vi "CreateCreepSamples2.vi"(0 "setValueForAESum":dbl, 5 "AEdataSum":dbl, 7 "outputLength":i32, 9 "changeOfForceWithinBufferLoop":dbl, 11 "initialOrPreviousForce":dbl) -> (8 "output array":dbl[][](array[numeric]))   [LabVIEW 2009]
panel:
  out "Number of points":i32=1000
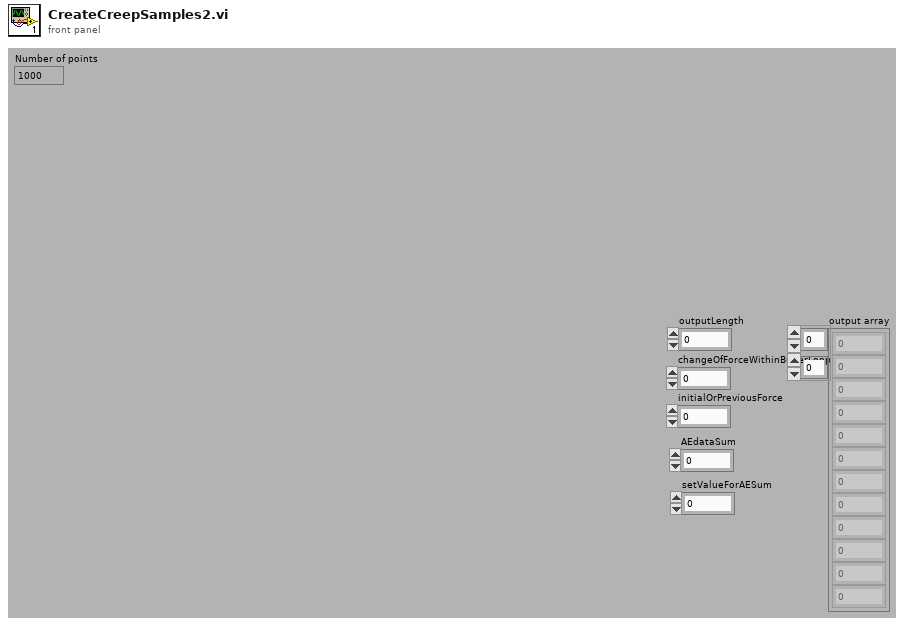
[diagram p1: front panel]
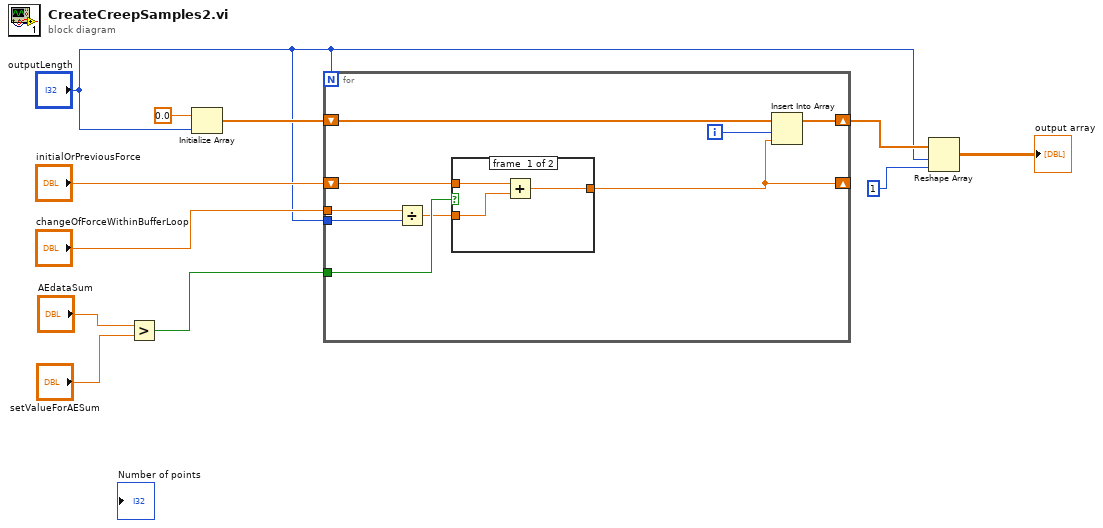
[diagram p0: block diagram]
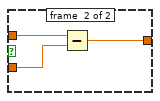
[diagram p2: hidden frame]
diagram:
  n1 = Greater?(x="AEdataSum", y="setValueForAESum") -> (0:w3:bool)
  n2 = Initialize Array(0.0 ("element"), "outputLength") -> (w8:dbl[])
  n3 = for {
    N: "outputLength" -> [_]
    shift-right: [w19] -> w7
    shift-left: w8 -> [w20]
    shift-right: [w12] -> _
    shift-left: "initialOrPreviousForce" -> [w14]
    tunnel: "changeOfForceWithinBufferLoop" -> [w17]
    tunnel: "outputLength" -> [w16]
    tunnel: w3 -> [w15]
    i -> [w18]
    n4 = Divide(x=w17, y=w16) -> (x/y=w13:dbl)
    n5 = case shown="True" w15 {
      tunnel: w14 -> [w23 w26]
      tunnel: w13 -> [w22 w25]
      tunnel: [w21 w24] -> w12
      frame #0 {
        n6 = Add(x=w23, y=w22) -> (x+y=w21:dbl)
      }
      frame #1 {
        n7 = Subtract(x=w26, y=w25) -> (x-y=w24:dbl)
      }
    }
    n8 = Insert Into Array(array=w20, index=w18, new element=w12) -> (w19:dbl[])
  }
  n9 = Reshape Array(w7, "outputLength", 1 ("dimension size")) -> (→"output array":dbl[][])
